vi "DN4_SetTimeOut.vi"(9 "error in (no error)":errorcluster, 10 "time out":i32, 11 "Task ID":u32) -> (1 "error out":errorcluster, 3 "Task ID":u32)   [LabVIEW 2009]
uses:
  Windows/System32/AdvLvDaq.dll
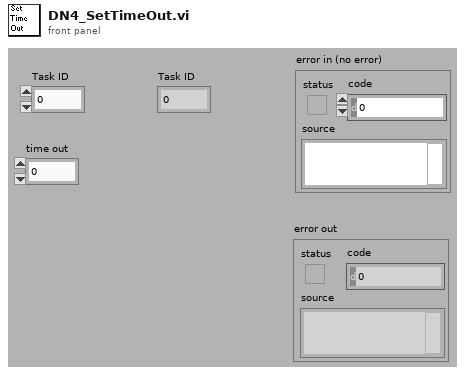
[diagram p1: front panel]
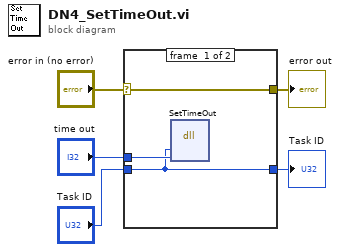
[diagram p0: block diagram]
diagram:
  n1 = case shown="No Error" "error in (no error)" {
    selector: "error in (no error)" -> [w6 w10]
    tunnel: "Task ID" -> [w7 w9]
    tunnel: "time out" -> [w8 _]
    tunnel: [w7 w9] -> w2
    tunnel: [w6 w10] -> w1
    frame #0 {
      n2 = dll-call lib="C:/Windows/System32/AdvLvDaq.dll" fn="SetTimeOut"("taskId"=w7, "timeout"=w8) -> ()  [unwired: 5 in, 3 out]
    }
    frame #1 {
    }
  }
  "Task ID" <- w2
  "error out" <- w1
